vi "Error_5113.vi"(8 "error in (no error)":errorcluster, 9 "Retry count":i32, 10 "Encoder":i32, 11 "Target Pos":i32) -> (0 "error out":errorcluster)   [LabVIEW 2015, in "Tool Module.lvlib"]
uses:
  Tool Module.lvlib
  <vilib>/Utility/error.llb/Error Cluster From Error Code.vi
  <vilib>/ErrorRing/Error Ring.xnode
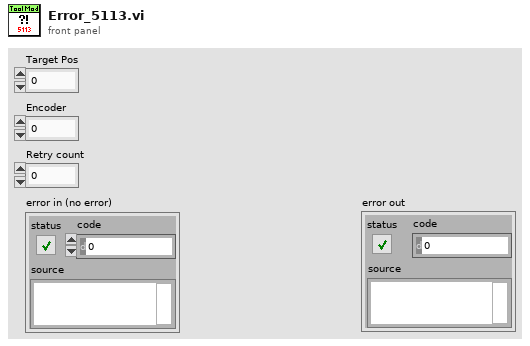
[diagram p1: front panel]
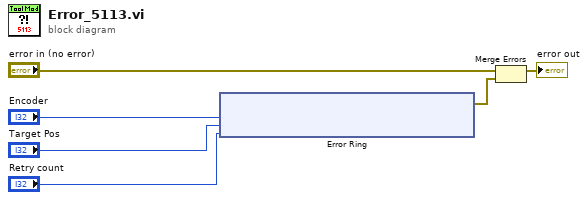
[diagram p0: block diagram]
diagram:
  n1 = xnode "Error Ring"("parameter 0"="Encoder", "parameter 1"="Target Pos", "parameter 2"="Retry count") -> ("error out"=w3:errorcluster)
  n2 = Merge Errors("error in (no error)", w3) -> (→"error out":errorcluster)
